vi "运维调试.vi"() -> ()   [LabVIEW 2016]
uses:
  <vilib>/Utility/miscctls.llb/LVPointTypeDef.ctl
  <vilib>/Utility/config.llb/NI_LVConfig.lvlib
panel:
  in  "运维调试菜单":enum16{"原位多参数", "集成式多参数", "营养盐"}(xcontrol)
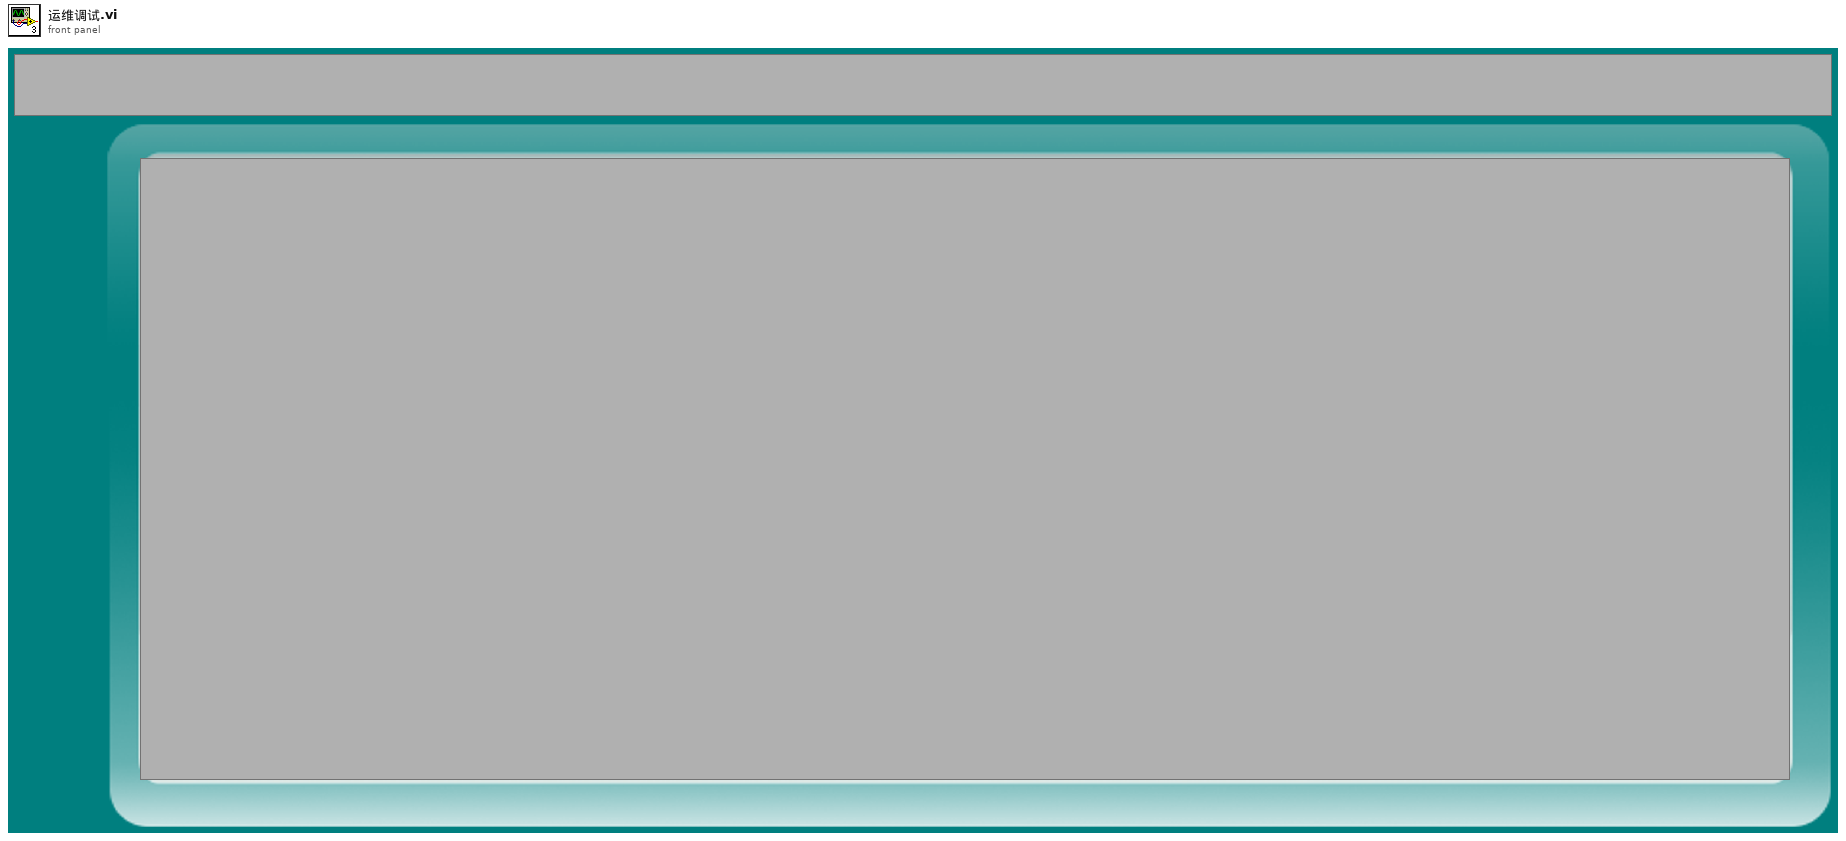
[diagram p1: front panel]
types:
  T1 = typedef "LVPointTypeDef.ctl" = cluster{"Horizontal":i16, "Vertical":i16}
  T2 = typedef "NI_LVConfig.lvlib/Config Data RefNum.ctl" = refnum<k1>
  T3 = enum32{"Bad", "Idle", "Run top level", "Running"}
  T4 = cluster{"集成式多参数":string, "营养盐":string, "原位多参数":string}
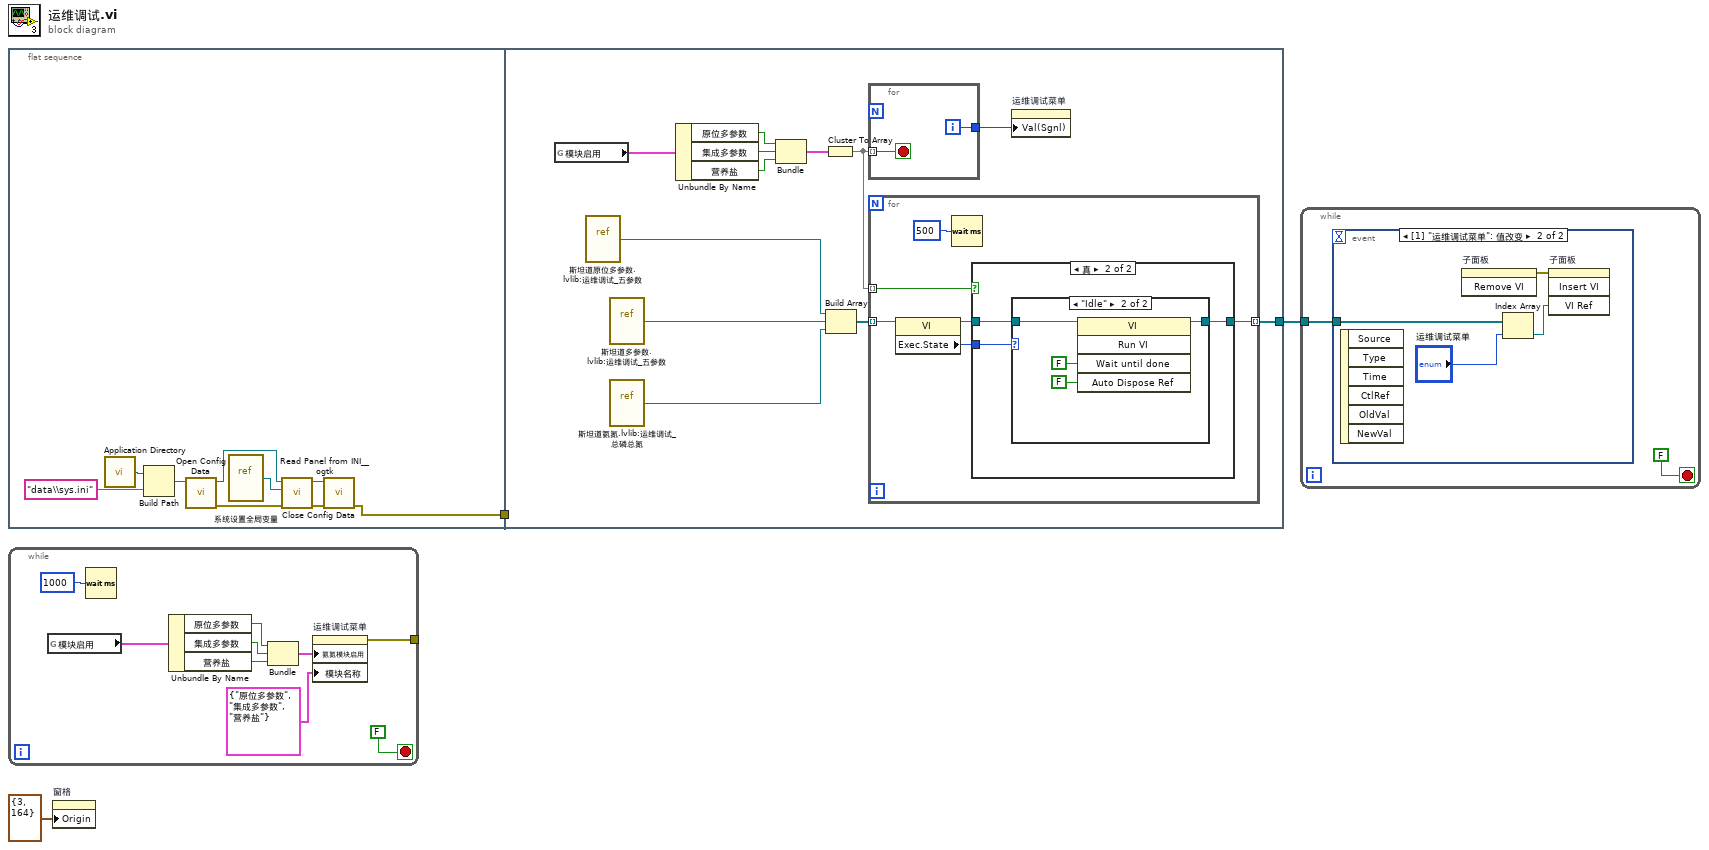
[diagram p0: block diagram]
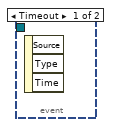
[diagram p4: hidden frame]
diagram:
  n1 = flat-sequence {
    tunnel: [w4] -> w1
    tunnel: w1 -> [_]
    tunnel: [w24] -> w2
    frame #0 {
      n2 = call <vilib>:"Application Directory.vi"() -> ("Application Directory"=w5:path)
      n3 = Build Path(base path=w5, name or relative path="data\\sys.ini" ("名称或相对路径")) -> (appended path=w7:path)
      n4 = call <vilib>:"Open Config Data.vi"("configuration file path"=w7) -> ("error out"=w11:errorcluster, "refnum"=w8:T2)  [unwired: 8 in, 1 out]
      n5 = vi-ref "系统设置全局变量.vi"() -> (w9:refnum<vi>)
      n6 = call <userlib>:"Read Panel from INI__ogtk.vi"("error in (no error)"=w11, "VI ref"=w9, "refnum"=w8) -> ("error out"=w12:errorcluster, "refnum out"=w10:T2)  [unwired: 7 in]
      n7 = call <vilib>:"Close Config Data.vi"("error in (no error)"=w12, "refnum"=w10) -> ("error out"=w4:errorcluster)  [unwired: 8 in, 1 out]
    }
    frame #1 {
      n8 = global read "系统设置全局变量.vi" "模块启用"() -> (w22:cluster{"原位多参数":bool, "集成多参数":bool, "营养盐":bool})
      n9 = vi-ref "斯坦道原位多参数.lvlib:运维调试_五参数.vi"() -> (w16:refnum<vi>)
      n10 = vi-ref "斯坦道多参数.lvlib:运维调试_五参数.vi"() -> (w15:refnum<vi>)
      n11 = vi-ref "斯坦道氨氮.lvlib:运维调试_总磷总氮.vi"() -> (w13:refnum<vi>)
      n12 = Unbundle By Name(w22) -> ("原位多参数"=w21:bool, "集成多参数"=w20:bool, "营养盐"=w14:bool)
      n13 = Bundle("原位多参数"=w21, "集成多参数"=w20, "营养盐"=w14) -> (w19:cluster{"原位多参数":bool, "集成多参数":bool, "营养盐":bool})  [unwired: 1 in]
      n14 = Cluster To Array(cluster=w19) -> (array=w18:bool[])
      n15 = Build Array(w16, w15, w13) -> (w23:refnum<vi>[])
      n16 = for {
        tunnel: w18 -> [w26] mode=indexing
        tunnel: [w25] -> w17
        i -> [w25]
        stop <- w26 stop-if-true
      }
      n17 = for {
        tunnel: w23 -> [w32] mode=indexing
        tunnel: [w31] -> w24 mode=indexing
        tunnel: w18 -> [w28] mode=indexing
        n18 = property class="VI"(reference=w32) -> (reference out=w29:refnum<vi>, "Exec.State"=w30:T3)  [unwired: 1 in, 1 out]
        n19 = Wait (ms)(milliseconds to wait=u32 500 ("等待时间（毫秒）")) -> ()  [unwired: 1 out]
        n20 = case shown="真" w28 {
          tunnel: [w33 w36] -> w31
          tunnel: w30 -> [_ w35]
          tunnel: w29 -> [w33 w34]
          frame False {
          }
          frame True {
            n21 = case shown="\"Idle\"" w35 {
              tunnel: w34 -> [w37 w39]
              tunnel: [w37 w38] -> w36
              frame "Bad", Default {
              }
              frame "Idle" {
                n22 = invoke class="VI" method="Run VI"(reference=w39, "Wait until done"=FALSE ("结束前等待"), "Auto Dispose Ref"=FALSE ("自动销毁引用")) -> (reference out=w38:refnum<vi>)  [unwired: 2 in, 4 out]
              }
            }
          }
        }
      }
      n23 = property on="运维调试菜单" class="运维调试菜单 (严格)"("Val(Sgnl)"=w17) -> ()  [unwired: 2 in, 2 out]
    }
  }
  n24 = while {
    tunnel: [w48] -> _
    stop <- FALSE stop-if-true
    n25 = global read "系统设置全局变量.vi" "模块启用"() -> (w47:cluster{"原位多参数":bool, "集成多参数":bool, "营养盐":bool})
    n26 = Wait (ms)(milliseconds to wait=u32 1000 ("等待时间（毫秒）")) -> ()  [unwired: 1 out]
    n27 = Unbundle By Name(w47) -> ("原位多参数"=w46:bool, "集成多参数"=w45:bool, "营养盐"=w44:bool)
    n28 = Bundle("原位多参数"=w46, "集成多参数"=w45, "营养盐"=w44) -> (w43:cluster{"原位多参数":bool, "集成多参数":bool, "营养盐":bool})  [unwired: 1 in]
    n29 = property on="运维调试菜单" class="运维调试菜单 (严格)"("氨氮模块启用"=w43, "模块名称"=T4 {"集成式多参数"="原位多参数", "营养盐"="集成多参数", "原位多参数"="营养盐"}) -> (error out=w48:errorcluster)  [unwired: 2 in, 1 out]
  }
  n30 = property on="窗格" class="Pane"("Origin"=T1 {"Horizontal"=3, "Vertical"=164} ("原点")) -> ()  [unwired: 2 in, 2 out]
  n31 = while {
    tunnel: w2 -> [w51]
    stop <- FALSE stop-if-true
    n32 = event shown="[1] \"运维调试菜单\": 值改变" {
      selector: _ -> [_ _]
      dyn-events: _ -> [_ _]
      timeout: _ -> [_ _]
      tunnel: w51 -> [_ w55]
      event Timeout {
        n33 = event-data() -> ()  [unwired: 1 in, 3 out]
      }
      event "运维调试菜单": Value Change {
        n34 = event-data() -> ()  [unwired: 1 in, 6 out]
        n35 = invoke on="子面板" class="SubPnl" method="Remove VI"() -> (error out=w56:errorcluster)  [unwired: 3 in, 2 out]
        n36 = Index Array(array=w55, index="运维调试菜单") -> (element=w54:refnum<vi>)
        n37 = invoke on="子面板" class="SubPnl" method="Insert VI"(error in=w56, "VI Ref"=w54) -> ()  [unwired: 2 in, 4 out]
      }
    }
  }
